vi "test AddGet Parameters Boolean.vi"(8 "error in (no error)":errorcluster, 11 "TestCase in":refnum<class "AddGet Parameters.lvclass">) -> (0 "error out":errorcluster, 3 "TestCase out":refnum<class "AddGet Parameters.lvclass">)   [LabVIEW 2018, in "AddGet Parameters.lvclass"]
uses:
  AddGet Parameters.lvclass
  Plugins/Utility/Test Classes/Test.lvclass
  <vilib>/Utility/Data Type/Type Definitions/Data Type.ctl
  <vilib>/addons/_JKI Toolkits/VI Tester/TestCase.llb/TestCase.lvclass
  <vilib>/Utility/Data Type/NI_Data Type.lvlib
  C:/Program Files (x86)/National Instruments/LabVIEW 2018/vi.lib/addons/_JKI Toolkits/VI Tester/TestCase.llb/TestCase.lvclass
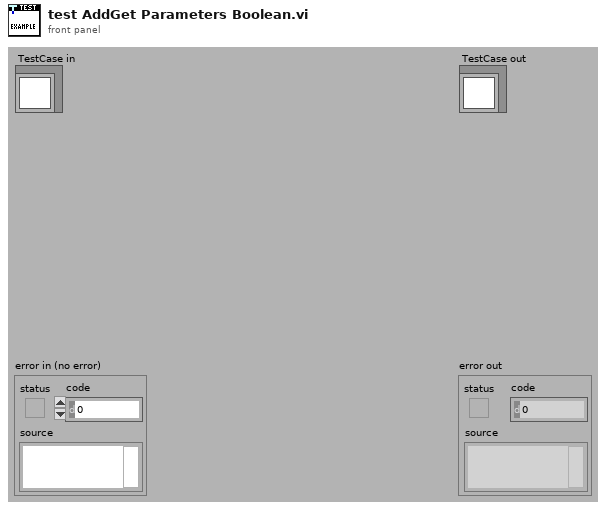
[diagram p1: front panel]
types:
  T1 = typedef "NI_Data Type.lvlib/Data Type.ctl" = enum8{"Invalid Type", "Void", "I8", "I16", "I32", "I64", "U8", "U16", "U32", "U64", "Single Float", "Double Float", "Extended Float", "Single Complex", "Double Complex", "Extended Complex", "Enum U8", "Enum U16", "Enum U32", "Enum U64", "Single Float With Unit", "Double Float With Unit", "Extended Float With Unit", "Single Complex with Unit", "Double Complex with Unit", "Extended Complex with Unit", "Boolean", "String", "Path", "Picture", "Tag", "Array", "Cluster", "Variant", "LV Variant", "Waveform", "Timestamp", "Digital Waveform", "Digital Data", "ExpressData", "Refnum", "External Data", "VI", "Poly VI", "LabVIEW Class Instance", "Fixed Point"}
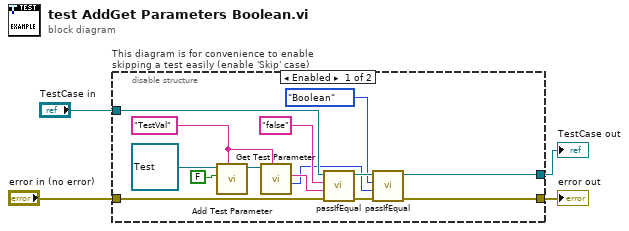
[diagram p0: block diagram]
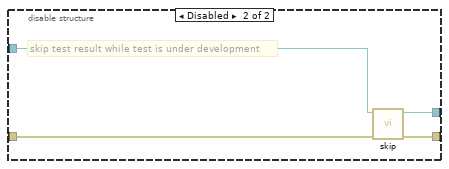
[diagram p2: hidden frame]
diagram:
  n1 = disable-structure "This diagram is for convenience to enable skipping a test easily (enable 'Skip' case)" shown="Enabled" {
    disable-tunnel: "TestCase in" -> [w18 w22]
    disable-tunnel: [w7 w20] -> w1
    disable-tunnel: [w9 w21] -> w3
    disable-tunnel: "error in (no error)" -> [w16 w19]
    frame Enabled {
      w12 = "TestVal" ("Data Value ID")
      n2 = call-dynamic "Add Test Parameter.vi"("Data Value ID"=w12, "Data Value"=FALSE, "Test in"=refnum<class "Test.lvclass"> refnum) -> ("Test out"=w13:refnum<class "Test.lvclass">)  [unwired: 6 in, 2 out]
      n3 = call "Get Test Parameter.vi"("Data Value ID"=w12, "Test in"=w13) -> ("Data Type"=w6:T1, "Test Parameter"=w11:string)  [unwired: 7 in, 1 out]
      n4 = call-dynamic "passIfEqual.vi"("error in (no error)"=w16, "y"=w11, "x"="false", "TestCase in"=w18) -> ("error out"=w17:errorcluster, "TestCase out"=w8:refnum<class "AddGet Parameters.lvclass">)  [unwired: 6 in]
      n5 = call-dynamic "passIfEqual.vi"("error in (no error)"=w17, "y"=w6, "x"=Data_Type."Boolean" ("Data Type"), "TestCase in"=w8) -> ("error out"=w9:errorcluster, "TestCase out"=w7:refnum<class "AddGet Parameters.lvclass">)  [unwired: 6 in]
    }
    frame Disabled {
      # "skip test result while test is under development"
      n6 = call <vilib>:"skip.vi"("error in (no error)"=w19, "TestCase in"=w22) -> ("error out"=w21:errorcluster, "TestCase out"=w20:refnum<class "AddGet Parameters.lvclass">)  [unwired: 8 in]
    }
  }
  "error out" <- w3
  "TestCase out" <- w1
